vi "dfd_DFXP_Double to DFXP (scaler).vi"(11 "Double":dbl format="%#_53g") -> (3 "FXP":T1={"value"=0, "wl"=0, "iwl"=0, "Signed"=TRUE} {"value" format="%.0x"})   [LabVIEW 2017, in "NI_DigFilter_FXP.lvlib"]
uses:
  <vilib>/addons/Digital Filter Design/NI_DigFilter_FXP.lvlib
  <vilib>/addons/Digital Filter Design/_Objects.llb/dfd_DFXP Data Type (scaler).ctl
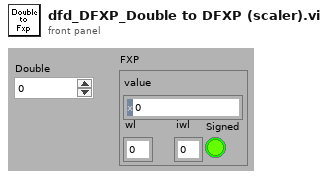
[diagram p1: front panel]
types:
  T1 = typedef "dfd_DFXP Data Type (scaler).ctl" = cluster{"value":i64, "wl":i16, "iwl":i16, "Signed":bool}
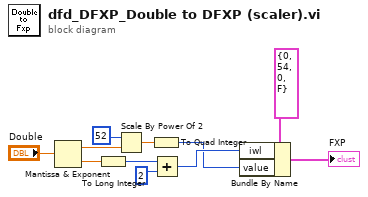
[diagram p0: block diagram]
diagram:
  n1 = Mantissa & Exponent(0:"Double") -> (1:w11:dbl, 2:w9:dbl)
  n2 = To Long Integer(number=w9) -> (32bit integer=w8:i32)
  n3 = Scale By Power Of 2(n=52, x=w11) -> (x*2^n=w6:dbl)
  n4 = To Quad Integer(1:w6) -> (0:w1:i64)
  n5 = Add(x=w8, y=2) -> (x+y=w4:i32)
  n6 = Bundle By Name(cluster=T1 {"value"=0, "wl"=54, "iwl"=0, "Signed"=FALSE} ("FXP"), "iwl"=w4, "value"=w1) -> (→"FXP":T1)
